vi "decodeCamerasReferee.vi"(8 "error in (no error)":errorcluster, 10 "element":u8[](array[numeric]), 11 "Vision in":refnum<class "Vision.lvclass">) -> (0 "error out":errorcluster, 2 "SSL Game Status":T1, 3 "Vision out":refnum<class "Vision.lvclass">)   [LabVIEW 2020, in "Vision.lvclass"]
uses:
  Vision.lvclass
  Old vision/Controls/SSL Referee.ctl
  Old vision/Decode SSL and Refree Wrapper Package Folder/SSL Referee Team Info.ctl
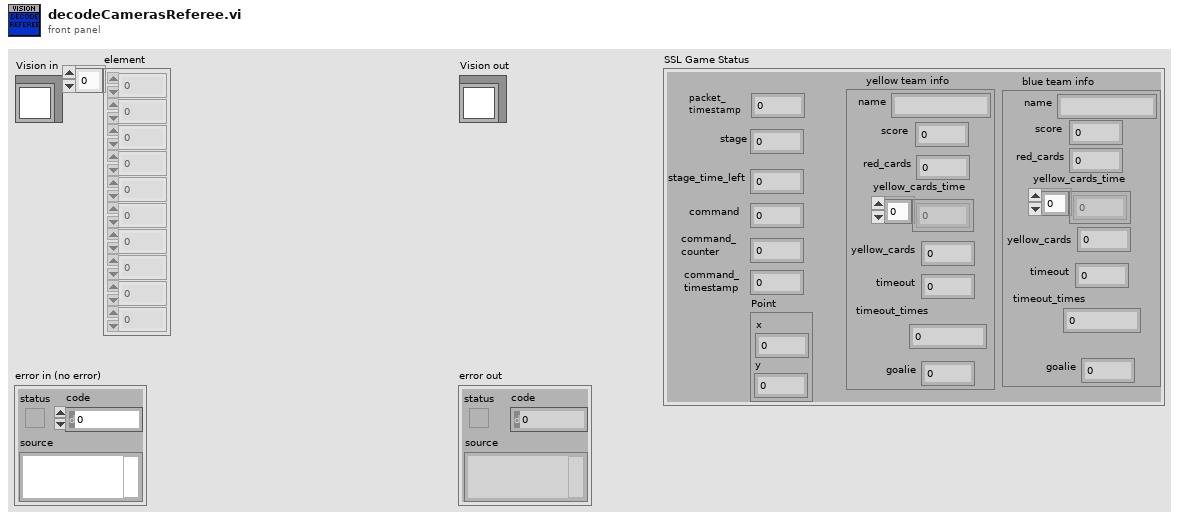
[diagram p1: front panel]
types:
  T1 = typedef "SSL Referee.ctl" = cluster{"packet_\ntimestamp":u64, "stage":u64, "stage_time_left":i32, "command ":u64, "command_\ncounter ":u32, "command_\ntimestamp":u64, "yellow team info":T2, "blue team info":T2, "Point":cluster{"x":sgl, "y":sgl}}
  T2 = typedef "SSL Referee Team Info.ctl" = cluster{"name":string, "score":u32, "red_cards":u32, "yellow_cards_time":u32[], "yellow_cards":u32, "timeout":u32, "timeout_times":u32, "goalie":u32}
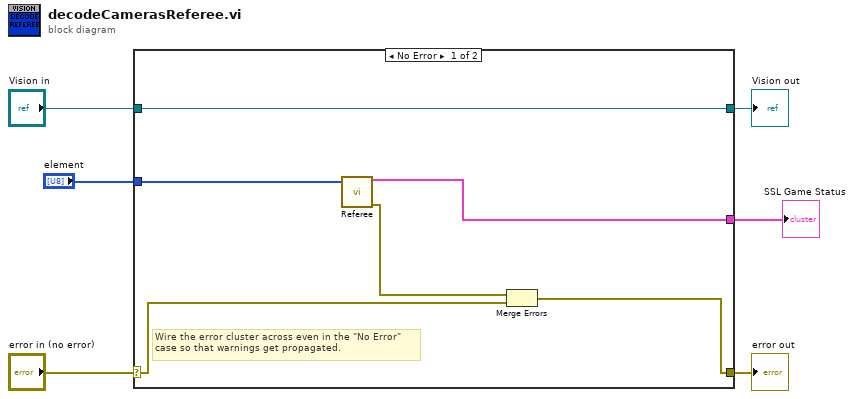
[diagram p0: block diagram]
diagram:
  n1 = case shown="No Error" "error in (no error)" {
    selector: "error in (no error)" -> [w8 w14]
    tunnel: [w7 w14] -> w5
    tunnel: [w12 w13] -> w3
    tunnel: "Vision in" -> [w12 w13]
    tunnel: "element" -> [w11 _]
    tunnel: [w10 _] -> w1
    frame No Error {
      # "Wire the error cluster across even in the \"No Error\"\ncase so that warnings get propagated."
      n2 = call "Referee.vi"("element"=w11) -> ("output cluster"=w10:T1, "error out"=w9:errorcluster)  [unwired: 13 in]
      n3 = Merge Errors(w9, w8) -> (w7:errorcluster)
    }
    frame Error {
    }
  }
  "error out" <- w5
  "Vision out" <- w3
  "SSL Game Status" <- w1
